vi "High Frequency Noise Cleaner.vi"(7 "Repeats":i32=10, 8 "Error In":errorcluster, 9 "Fractional Damping":dbl=0.4, 10 "Fractional Threshold":dbl=0.1, 11 "Array in":dbl[](array[numeric])) -> (0 "Error Out":errorcluster, 3 "Array out":dbl[](array[numeric]))   [LabVIEW 2021, in "Math.lvlib"]
uses:
  71ed2770-aab7-4d60-a307-3f9f1393e19b.vi
  040261d9-0997-4b8d-9ff3-e1923cd8371a.vi
  Arrays/Signed Array Index.vi
  Math.lvlib
panel:
  # "see the License on the block diagram (Ctrl+E or Window:Show Block Diagram)"
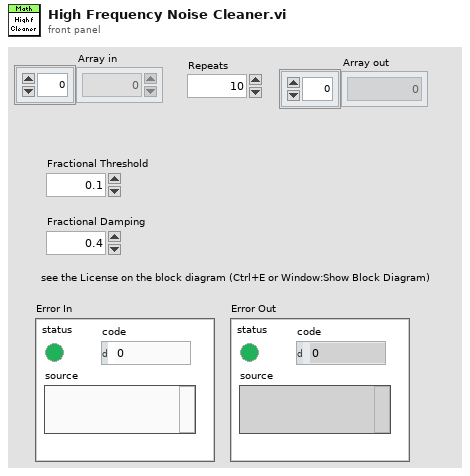
[diagram p1: front panel]
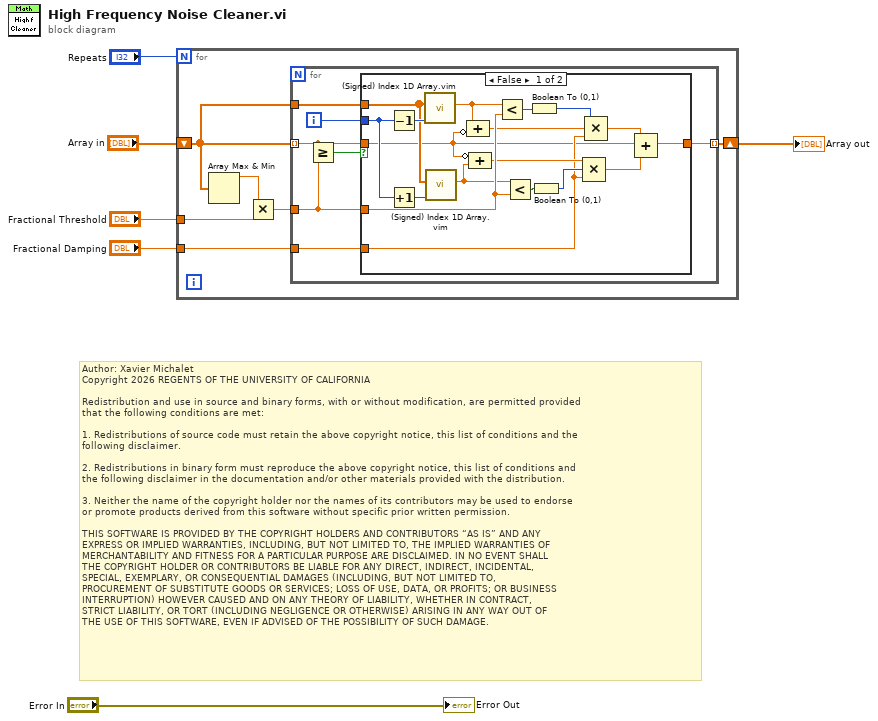
[diagram p0: block diagram]
diagram:
  # "Author: Xavier Michalet\nCopyright 2026 REGENTS OF THE UNIVERSITY OF CALIFORNIA\n\nRedistribution and use in source and binary forms, with or without modification, are permitted provided\nthat the following conditions are met:\n\n1. Redistributions of source code must retain the above copyright notice, this list of conditions and the\nfollowing disclaimer.\n\n2. Redistributions in binary form must reproduce the above copyright notice, this list of conditions and\nthe following disclaimer in the documentation and/or other materials provided with the distribution.\n\n3. Neither the name of the copyright holder nor the names of its contributors may be used to endorse \nor promote products derived from this software without specific prior written permission.\n\nTHIS SOFTWARE IS PROVIDED BY THE COPYRIGHT HOLDERS AND CONTRIBUTORS “AS IS” AND ANY \nEXPRESS OR IMPLIED WARRANTIES, INCLUDING, BUT NOT LIMITED TO, THE IMPLIED WARRANTIES OF\nMERCHANTABILITY AND FITNESS FOR A PARTICULAR PURPOSE ARE DISCLAIMED. IN NO EVENT SHALL\nTHE COPYRIGHT HOLDER OR CONTRIBUTORS BE LIABLE FOR ANY DIRECT, INDIRECT, INCIDENTAL, \nSPECIAL, EXEMPLARY, OR CONSEQUENTIAL DAMAGES (INCLUDING, BUT NOT LIMITED TO, \nPROCUREMENT OF SUBSTITUTE GOODS OR SERVICES; LOSS OF USE, DATA, OR PROFITS; OR BUSINESS\nINTERRUPTION) HOWEVER CAUSED AND ON ANY THEORY OF LIABILITY, WHETHER IN CONTRACT, \nSTRICT LIABILITY, OR TORT (INCLUDING NEGLIGENCE OR OTHERWISE) ARISING IN ANY WAY OUT OF\nTHE USE OF THIS SOFTWARE, EVEN IF ADVISED OF THE POSSIBILITY OF SUCH DAMAGE."
  n1 = for {
    N: "Repeats" -> [_]
    tunnel: "Fractional Threshold" -> [w10]
    tunnel: "Fractional Damping" -> [w7]
    shift-right: [w8] -> w4
    shift-left: "Array in" -> [w12]
    n2 = Array Max & Min(array=w12) -> (max value=w11:dbl)  [unwired: 3 out]
    n3 = Multiply(x=w11, y=w10) -> (x*y=w9:dbl)
    n4 = for {
      tunnel: w12 -> [w16] mode=indexing
      tunnel: w12 -> [w18]
      tunnel: w9 -> [w14]
      tunnel: [w15] -> w8 mode=indexing
      tunnel: w7 -> [w13]
      i -> [w19]
      n5 = Greater Or Equal?(x=w16, y=w14) -> (x >= y?=w17:bool)
      n6 = case shown="False" w17 {
        tunnel: w19 -> [w36 _]
        tunnel: w18 -> [w35 _]
        tunnel: w16 -> [w22 w38]
        tunnel: [w20 w38] -> w15
        tunnel: w14 -> [w33 _]
        tunnel: w13 -> [w24 _]
        frame False {
          n7 = Decrement(x=w36) -> (x-1=w37:i32)
          n8 = Increment(x=w36) -> (x+1=w34:i32)
          n9 = call "(Signed) Index 1D Array.vim"("Signed Index"=w37, "Array"=w35) -> ("Array Element"=w32:dbl)  [unwired: 9 in]
          n10 = call "(Signed) Index 1D Array.vim"("Signed Index"=w34, "Array"=w35) -> ("Array Element"=w31:dbl)  [unwired: 9 in]
          n11 = Compound Arithmetic op=ADD(w32, invert w22) -> (w28:dbl)
          n12 = Compound Arithmetic op=ADD(invert w22, w31) -> (w26:dbl)
          n13 = Less?(x=w32, y=w33) -> (x < y?=w30:bool)
          n14 = Less?(x=w31, y=w33) -> (x < y?=w29:bool)
          n15 = Boolean To (0,1)(Boolean=w30) -> (0, 1=w27:i16)
          n16 = Boolean To (0,1)(Boolean=w29) -> (0, 1=w25:i16)
          n17 = Compound Arithmetic op=MULTIPLY(w26, w25, w24) -> (w21:dbl)
          n18 = Compound Arithmetic op=MULTIPLY(w27, w28, w24) -> (w23:dbl)
          n19 = Compound Arithmetic op=ADD(w23, w22, w21) -> (w20:dbl)
        }
        frame True {
        }
      }
    }
  }
  "Array out" <- w4
  "Error Out" <- "Error In"
